vi "圆环ROI转双矩形.vi"(11 "Annulus 2":T2={"Center X"=1245, "Center Y"=1480, "Inner Radius"=238, "Outer Radius"=308, "Start Angle"=0.0, "End Angle"=0.0} {"End Angle" min=-90.0 max=90.0 step=1.0 format="%.2f"; "Start Angle" min=-90.0 max=90.0 step=1.0 format="%.2f"; "Center X" scale=0.0..1024.0}) -> (2 "内环":T1, 3 "外环":T1)   [LabVIEW 2017]
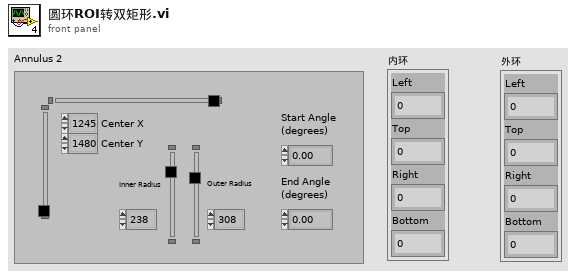
[diagram p1: front panel]
types:
  T1 = cluster{"Left":i32, "Top":i32, "Right":i32, "Bottom":i32}
  T2 = typedef "IMAQ Circle" = cluster{"Center X":i32, "Center Y":i32, "Inner Radius":i32, "Outer Radius":i32, "Start Angle":dbl, "End Angle":dbl}
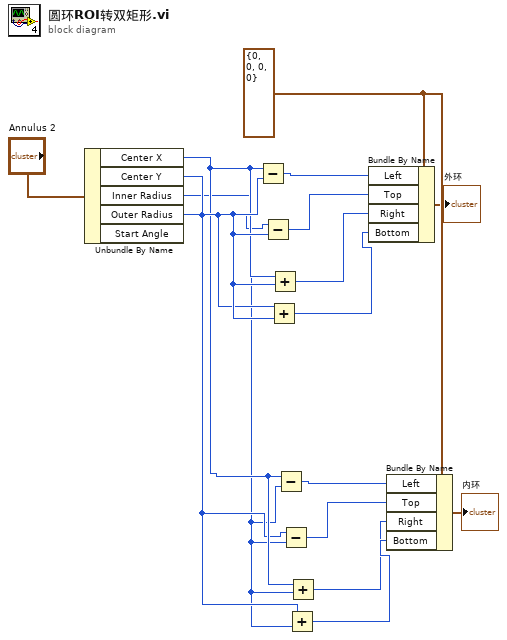
[diagram p0: block diagram]
diagram:
  w6 = T1 {"Left"=0, "Top"=0, "Right"=0, "Bottom"=0} ("Rectangle")
  n1 = Unbundle By Name("Annulus 2") -> ("Center X"=w5:i32, "Center Y"=w4:i32, "Inner Radius"=w3:i32, "Outer Radius"=w13:i32)  [unwired: 1 out]
  n2 = Subtract(x=w5, y=w13) -> (x-y=w15:i32)
  n3 = Subtract(x=w4, y=w13) -> (x-y=w14:i32)
  n4 = Add(x=w4, y=w13) -> (x+y=w11:i32)
  n5 = Add(x=w5, y=w13) -> (x+y=w12:i32)
  n6 = Subtract(x=w5, y=w3) -> (x-y=w7:i32)
  n7 = Subtract(x=w4, y=w3) -> (x-y=w8:i32)
  n8 = Add(x=w4, y=w3) -> (x+y=w10:i32)
  n9 = Add(x=w5, y=w3) -> (x+y=w9:i32)
  n10 = Bundle By Name(cluster=w6, "Left"=w15, "Top"=w14, "Right"=w12, "Bottom"=w11) -> (→"外环":T1)
  n11 = Bundle By Name(cluster=w6, "Left"=w7, "Top"=w8, "Right"=w9, "Bottom"=w10) -> (→"内环":T1)
